vi "12-QNET_MECHKIT_Switch_Debounce.vi"() -> ()   [LabVIEW 2012]
doc: "This VI is to be used with the NI-ELVIS and the QNET-Mechatronic Sensors I module. The objective is to examine the debounce in the micro switch and push button."
panel:
  in  "Trigger":T1={"Trigger Source"=1, "Trigger Type"=0, "Slope"=0, "Level (V)"=0.0, "Horizontal Position"=50} {"Slope" items=["Positive", "Negative"]; "Trigger Type" items=["Edge", "Digital", "Immediate"]; "Trigger Source" items=["TRIG"=0, "SYNC"=3, "Chan 0 Source"=1, "Chan 1 Source"=2]}
  out "Micro Switch":dynamicdata(graph) caption="Micro Switch / ELVIS Ch0"
  out "Push Button":dynamicdata(graph) caption="Push Button / ELVIS Ch1"
  in  "Dev":tag="Dev1"
  # "QNET-MECHKIT Debounce"
  # "NOTE: Place J8 jumper on \"Micro Switch\" and J9 on \"Push Button\"."
  # "1) Setup the Trigger below for micro switch (ELVIS Ch0) or \npush button (ELVIS Ch1).\n2) Run the VI.\n3) Press on either the micro switch or push button. VI should stop\nand generate a response in the graphs."
  # "s"
  # "Trigger"
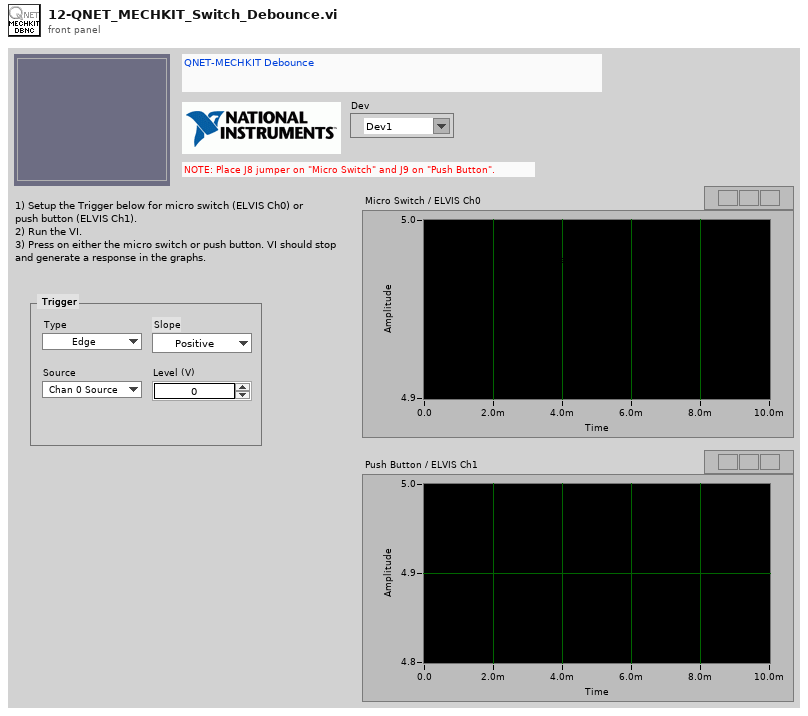
[diagram p1: front panel]
types:
  T1 = cluster{"Trigger Source":u16, "Trigger Type":u16, "Slope":i32, "Level (V)":dbl, "Horizontal Position":i32}
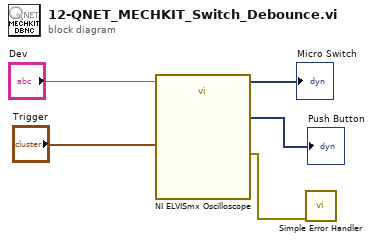
[diagram p0: block diagram]
diagram:
  n1 = call "NI ELVISmx Oscilloscope"("Device Name"="Dev", "Trigger"="Trigger") -> ("ELVIS/Channel 0"=→"Micro Switch":dynamicdata, "ELVIS/Channel 1"=→"Push Button":dynamicdata, "error out"=w2:errorcluster)  [unwired: 7 in, 8 out]
  n2 = call <vilib>:"Simple Error Handler.vi"("error in (no error)"=w2) -> ()  [unwired: 1 in, 8 out]
